vi "DMC VIDoc Confluence.vi"(8 "Error in":errorcluster caption="Error in (no error)") -> ()   [LabVIEW 2023]
uses:
  Git Type.ctl
  DMC CLI Confluence Documentation State.ctl
  <vilib>/Wiresmith Technology/G CLI/CLI Class/CLI.lvclass
  <vilib>/DMC/VIDoc/Printers/Confluence/Confluence Printer/Types/File Change Map.ctl
  Confluence Settings.ctl
  <vilib>/DMC/VIDoc/Framework/Parsing/TypeDefs/Full Documentation Info.ctl
  <vilib>/DMC/VIDoc/Framework/Parsing/Project Documentation/Project Documentation.lvclass
  <vilib>/DMC/VIDoc/Framework/Parsing/Interface Documenation/Interface Documenation.lvclass
  <vilib>/DMC/VIDoc/Framework/Parsing/Class Documentation/Class Documentation.lvclass
  <vilib>/DMC/VIDoc/Framework/Parsing/Library Documentation/Library Documentation.lvclass
  <vilib>/DMC/VIDoc/Framework/Parsing/GUI Documentation/GUI Documentation.lvclass
  <vilib>/DMC/VIDoc/Framework/Parsing/LLB Documentation/LLB Documentation.lvclass
  <vilib>/Wiresmith Technology/G CLI/Argument Parser/Option Class/Option Configuration.ctl
  <vilib>/Wiresmith Technology/G CLI/Argument Parser/Option Class/Argument Type.ctl
  8042783b-93c0-44c7-9b89-4fb89b10c9de.vi
  g-CLI Interaction/g-CLI Interaction.lvclass
  C:/Program Files/National Instruments/LabVIEW 2023/vi.lib/DMC/VIDoc/Framework/UI Interaction/Interface/UI Interaction.lvclass
  <vilib>/DMC/VIDoc/Printers/Confluence/Confluence Printer/VIDoc Printer - Confluence.lvclass
  <vilib>/Wiresmith Technology/G CLI/Argument Parser/Option Set Class/Option Set.lvclass
  <vilib>/Wiresmith Technology/G CLI/Argument Parser/Option Class/Option.lvclass
  <vilib>/DMC/VIDoc/Framework/Parsing/Documentation Parser/VIDoc Parser.lvclass
  <vilib>/DMC/VIDoc/Framework/Parsing/VIDoc Parsing.lvlib
panel:
  out "Scoped Token?":bool
  out "Confluence Token":string
  out "Confluence Email":string
  out "Confluence URL":string
  out "Use Data Center for Confluence Connection?":bool
  out "Use Login INI file for Confluence Connection?":bool
  out "Use Settings file for Confluence Connection Settings?":bool
  out "Top Page ID":string
  out "Source Paths":path[](array[path])
  out "Git Type":T1
  out "Run Git History?":bool
  out "Doc Settings Path":path
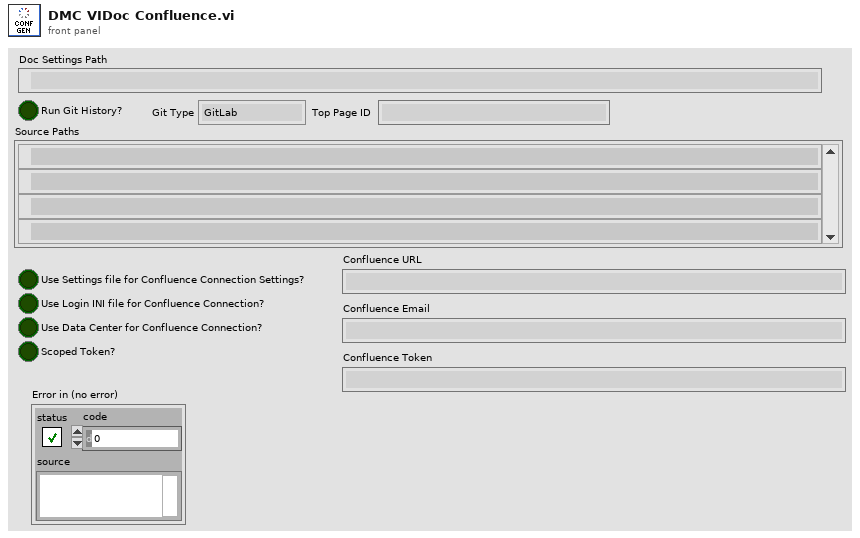
[diagram p1: front panel]
types:
  T1 = typedef "Git Type.ctl" = enum16{"GitLab", "GitHub", "BitBucket"}
  T2 = typedef "VIDoc Printer - Confluence.lvlib/VIDoc Printer - Confluence.lvclass/File Change Map.ctl" = map{string, cluster{"Timestamp":timestamp, "Commit Hash":string, "Author Name":string, "Branch":string, "Commit Hash URL":string}}
  T3 = typedef "Confluence Settings.ctl" = cluster{"Use INI?":bool, "URL":string, "Email":string, "Token":string, "Use Settings File?":bool, "Data Center?":bool, "Scoped Token?":bool}
  T4 = typedef "VIDoc Parsing.lvlib/Full Documentation Info.ctl" = cluster{"Projects":refnum<class "Project Documentation.lvclass">[], "Interfaces":refnum<class "Interface Documenation.lvclass">[], "Classes":refnum<class "Class Documentation.lvclass">[], "Libraries":refnum<class "Library Documentation.lvclass">[], "VI Members":refnum<class "GUI Documentation.lvclass">[], "Controls":refnum<class "GUI Documentation.lvclass">[], "LLBs":refnum<class "LLB Documentation.lvclass">[], "Bookmarked Map":map{string, refnum<class "GUI Documentation.lvclass">[]}}
  T5 = cluster{"CLI":refnum<class "CLI.lvclass">, "Working Directory":path, "Doc Settings Path":path, "Git History?":bool, "Git Type":T1, "File Change Map":T2, "Source Paths":path[], "Top Page ID":string, "Confluence Settings":T3, "Full Documentation":T4}
  T6 = typedef "DMC CLI Confluence Documentation State.ctl" = enum16{"Initialize", "Display Settings", "Git History", "Fetch Documentation", "Create Documentation", "Close", "Help"}
  T7 = enum16{"Doc Settings Path", "Git History", "Git Type", "Source Rel Paths", "Top Page ID", "Confluence Use Settings", "Confluence Use INI", "Confluence Type", "Confluence URL", "Confluence Email", "Confluence Token", "Scoped Token"}
  T8 = typedef "Option Parser.lvlib/Option.lvclass/Option Configuration.ctl" = cluster{"Option Type":T9, "Option Labels":string[], "Key":string, "Description":string, "Required":bool, "Default Value":string}
  T9 = typedef "Option Parser.lvlib/Option.lvclass/Argument Type.ctl" = enum16{"flag", "value"}
  T10 = enum16{"Doc Settings Path", "Git History", "Git Type", "Source Rel Paths", "Top Page ID", "Confluence Use Settings", "Confluence Use INI", "Confluence Type", "Confluence URL", "Confluence Email", "Confluence Token", "Scoped Token"}[]
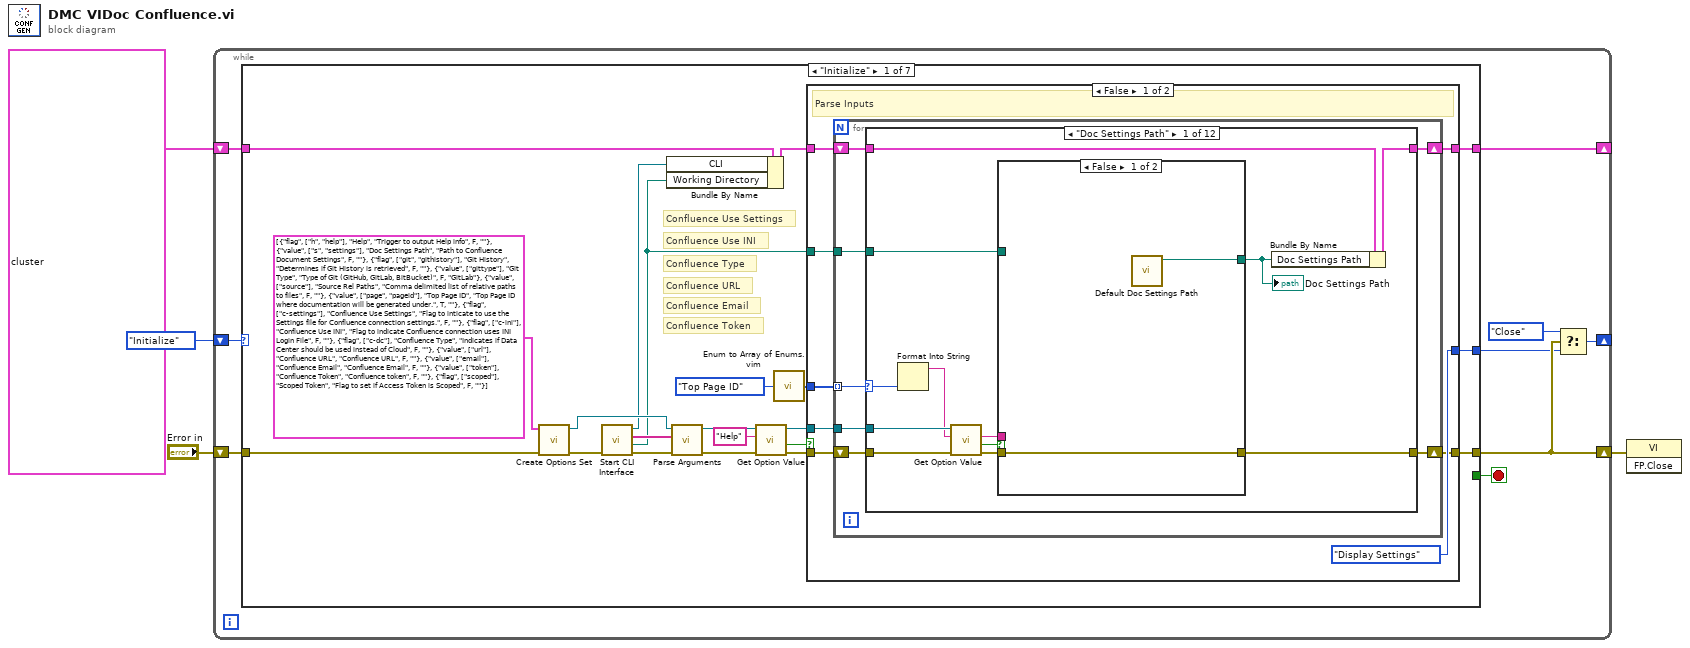
[diagram p0: block diagram]
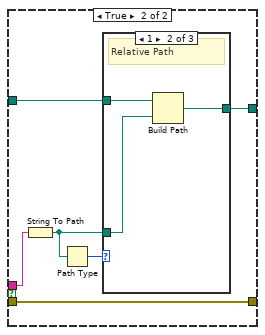
[diagram p2: hidden frame]
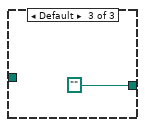
[diagram p4: hidden frame]
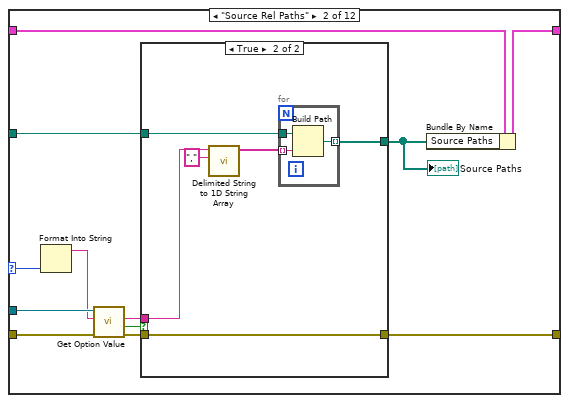
[diagram p5: hidden frame]
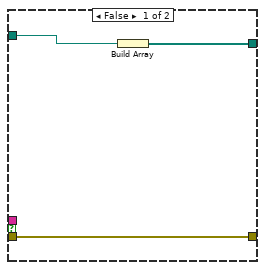
[diagram p6: hidden frame]
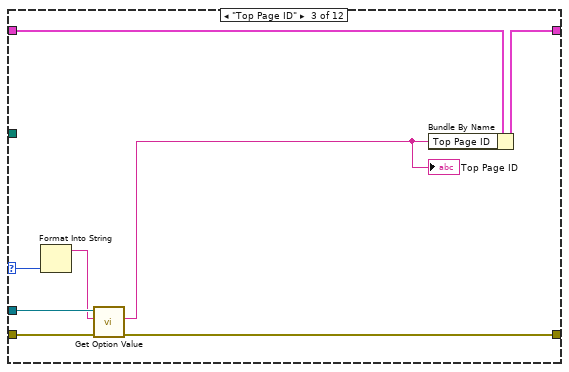
[diagram p7: hidden frame]
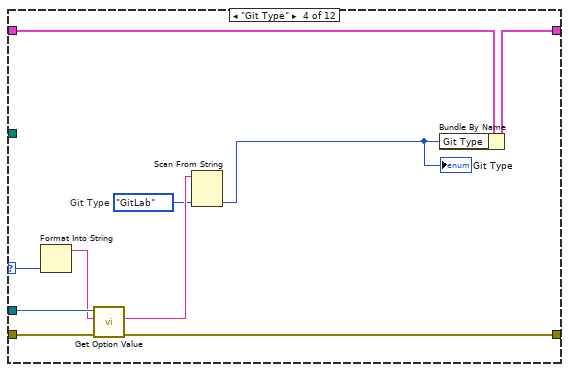
[diagram p8: hidden frame]
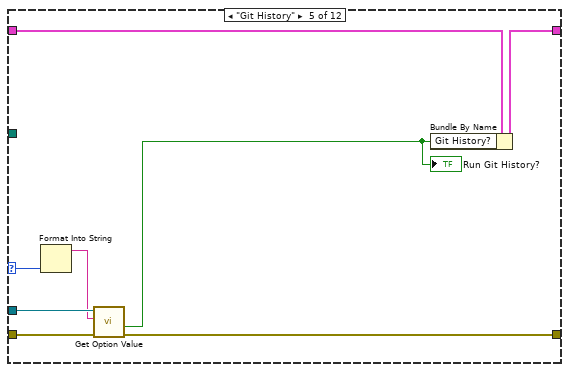
[diagram p9: hidden frame]
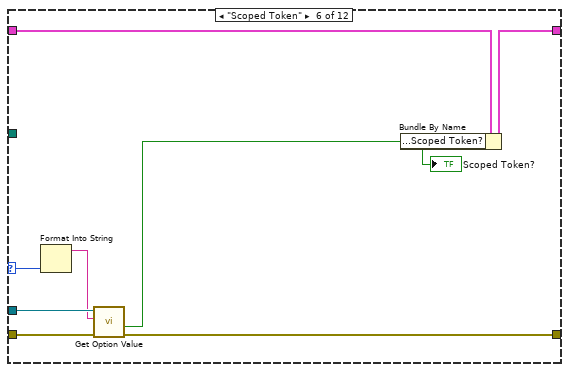
[diagram p10: hidden frame]
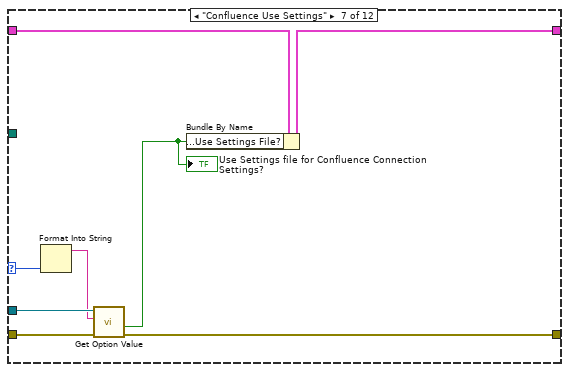
[diagram p11: hidden frame]
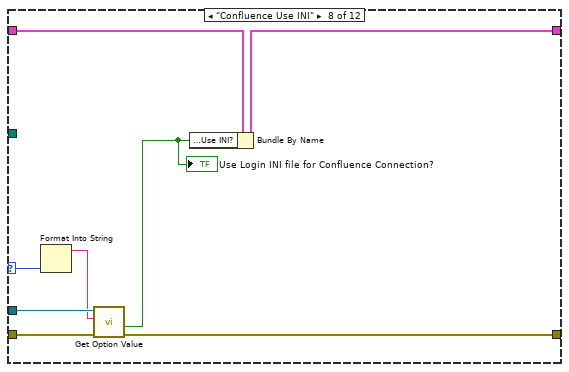
[diagram p12: hidden frame]
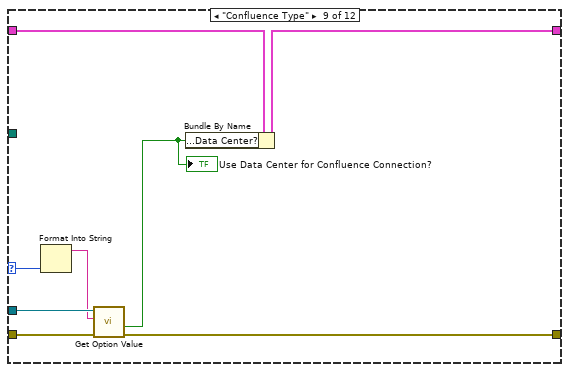
[diagram p13: hidden frame]
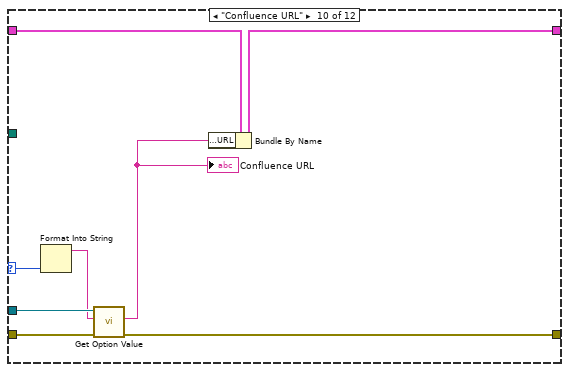
[diagram p14: hidden frame]
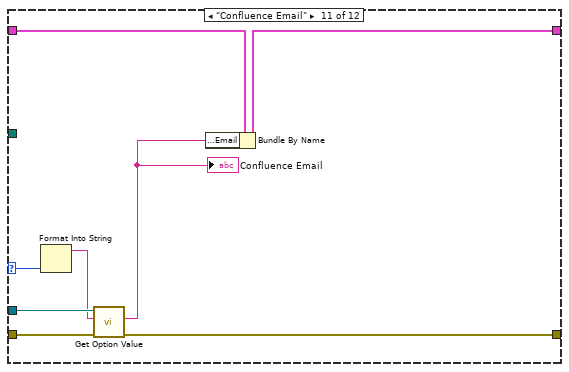
[diagram p15: hidden frame]
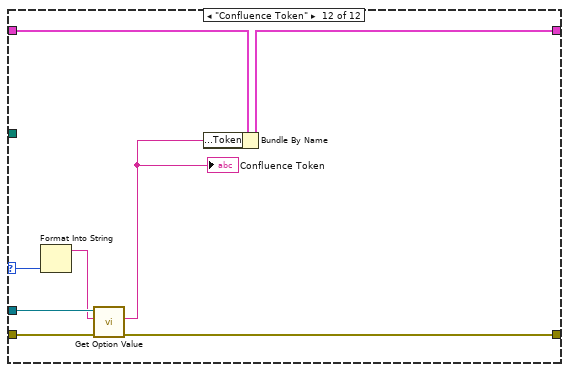
[diagram p16: hidden frame]
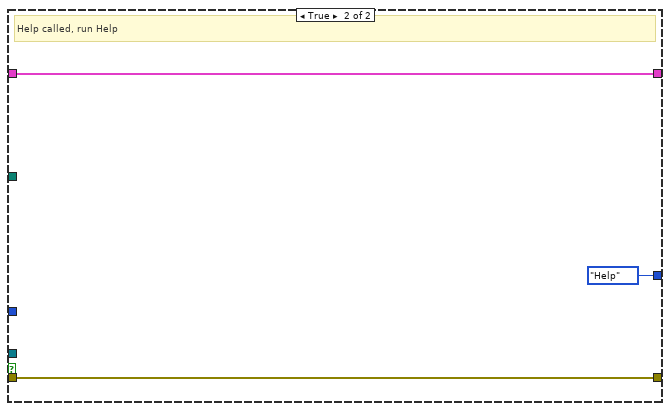
[diagram p17: hidden frame]
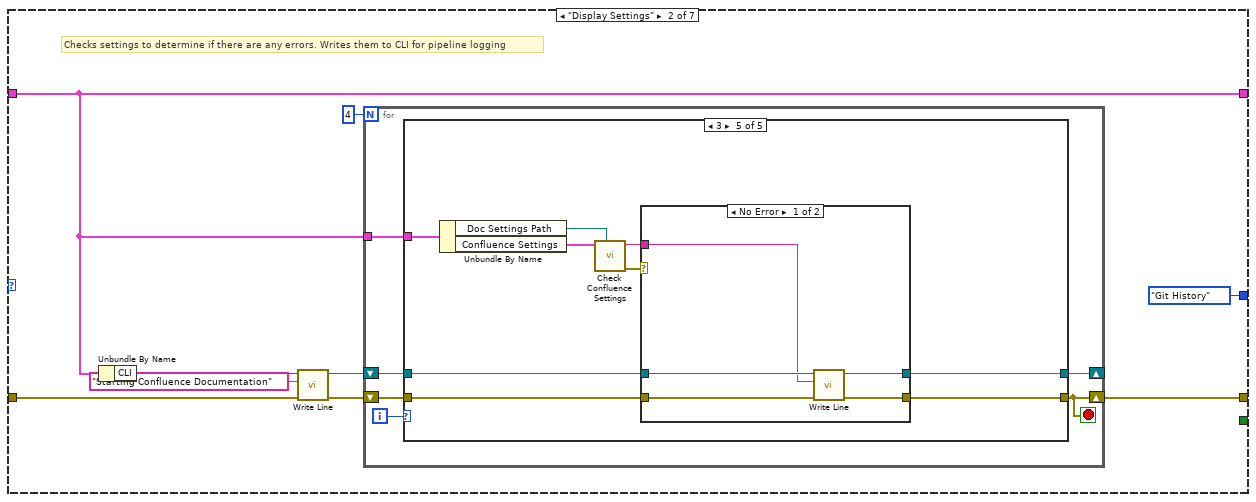
[diagram p18: hidden frame]
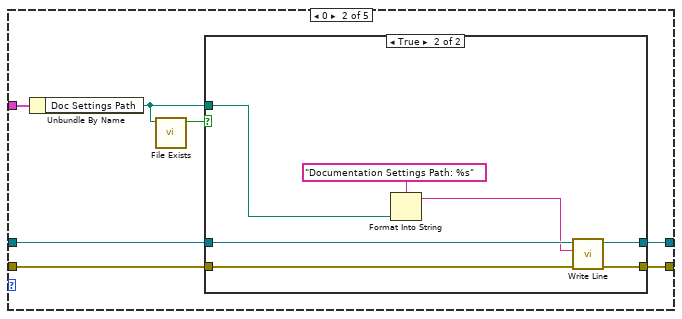
[diagram p20: hidden frame]
diagram:
  n1 = while {
    shift-right: [w8] -> _
    shift-left: DMC_CLI_Confluence_Documentation_State."Initialize" -> [w13]
    shift-right: [w10] -> w1
    shift-left: "Error in" -> [w12]
    shift-right: [w5] -> _
    shift-left: T5 {"CLI"=refnum, "Working Directory"=path "", "Doc Settings Path"=path "", "Git History?"=FALSE, "Git Type"=enum."GitLab", "File Change Map"={}, "Source Paths"=[], "Top Page ID"="", "Confluence Settings"={"Use INI?"=FALSE, "URL"="", "Email"="", "Token"="", "Use Settings File?"=FALSE, "Data Center?"=FALSE, "Scoped Token?"=FALSE}, "Full Documentation"={"Projects"=[], "Interfaces"=[], "Classes"=[], "Libraries"=[], "VI Members"=[], "Controls"=[], "LLBs"=[], "Bookmarked Map"={}}} -> [w6]
    stop <- w7 stop-if-true
    n2 = case shown="\"Initialize\"" w13 {
      tunnel: w12 -> [w26 w187 w272 w308 w322 w334 w344]
      tunnel: [w17 w192 w269 w292 w324 w335 w345] -> w10
      tunnel: [w19 DMC_CLI_Confluence_Documentation_State."Git History" DMC_CLI_Confluence_Documentation_State."Fetch Documentation" DMC_CLI_Confluence_Documentation_State."Create Documentation" DMC_CLI_Confluence_Documentation_State."Close" DMC_CLI_Confluence_Documentation_State."Close" DMC_CLI_Confluence_Documentation_State."Close"] -> w9
      tunnel: [_ _ _ _ _ TRUE _] -> w7
      tunnel: w6 -> [w25 w191 w270 w309 w323 w338 w342]
      tunnel: [w21 w191 w271 w303 w323 w338 w342] -> w5
      frame "Initialize" {
        # "Confluence Token"
        # "Confluence Email"
        # "Confluence URL"
        # "Confluence Type"
        # "Confluence Use INI"
        # "Confluence Use Settings"
        n3 = call <vilib>:"Create Options Set.vi"("error in (no error)"=w26, "Options"=T8[] [{"Option Type"=enum."flag", "Option Labels"=["h", "help"], "Key"="Help", "Description"="Trigger to output Help info", "Required"=FALSE, "Default Value"=""}, {"Option Type"=enum."value", "Option Labels"=["s", "settings"], "Key"="Doc Settings Path", "Description"="Path to Confluence Document Settings", "Required"=FALSE, "Default Value"=""}, {"Option Type"=enum."flag", "Option Labels"=["git", "githistory"], "Key"="Git History", "Description"="Determines if Git History is retrieved", "Required"=FALSE, "Default Value"=""}, {"Option Type"=enum."value", "Option Labels"=["gittype"], "Key"="Git Type", "Description"="Type of Git (GitHub, GitLab, BitBucket)", "Required"=FALSE, "Default Value"="GitLab"}, {"Option Type"=enum."value", "Option Labels"=["source"], "Key"="Source Rel Paths", "Description"="Comma delimited list of relative paths to files", "Required"=FALSE, "Default Value"=""}, {"Option Type"=enum."value", "Option Labels"=["page", "pageid"], "Key"="Top Page ID", "Description"="Top Page ID where documentation will be generated under.", "Required"=TRUE, "Default Value"=""}, {"Option Type"=enum."flag", "Option Labels"=["c-settings"], "Key"="Confluence Use Settings", "Description"="Flag to inticate to use the Settings file for Confluence connection settings.", "Required"=FALSE, "Default Value"=""}, {"Option Type"=enum."flag", "Option Labels"=["c-ini"], "Key"="Confluence Use INI", "Description"="Flag to indicate Confluence connection uses INI Login File", "Required"=FALSE, "Default Value"=""}, {"Option Type"=enum."flag", "Option Labels"=["c-dc"], "Key"="Confluence Type", "Description"="Indicates if Data Center should be used instead of Cloud", "Required"=FALSE, "Default Value"=""}, {"Option Type"=enum."value", "Option Labels"=["url"], "Key"="Confluence URL", "Description"="Confluence URL", "Required"=FALSE, "Default Value"=""}, {"Option Type"=enum."value", "Option Labels"=["email"], "Key"="Confluence Email", "Description"="Confluence Email", "Required"=FALSE, "Default Value"=""}, {"Option Type"=enum."value", "Option Labels"=["token"], "Key"="Confluence Token", "Description"="Confluence token", "Required"=FALSE, "Default Value"=""}, {"Option Type"=enum."flag", "Option Labels"=["scoped"], "Key"="Scoped Token", "Description"="Flag to set if Access Token is Scoped", "Required"=FALSE, "Default Value"=""}]) -> ("error out"=w32:errorcluster, "Option Set out"=w31:refnum<class "Option Set.lvclass">)  [unwired: 8 in]
        n4 = call <vilib>:"Start CLI Interface.vi"("error in (no error)"=w32) -> ("error out"=w34:errorcluster, "Working Directory"=w14:path, "Custom Parameters"=w30:string[], "CLI out"=w24:refnum<class "CLI.lvclass">)  [unwired: 7 in]
        n5 = Bundle By Name(cluster=w25, "CLI"=w24, "Working Directory"=w14) -> (w20:T5)
        n6 = call <vilib>:"Parse Arguments.vi"("error in (no error)"=w34, "Arguments"=w30, "Option Set in"=w31) -> ("error out"=w28:errorcluster, "Option Set out"=w27:refnum<class "Option Set.lvclass">)  [unwired: 5 in, 2 out]
        n7 = call <vilib>:"Get Option Value.vi"("error in (no error)"=w28, "Option Key"="Help", "Option Set in"=w27) -> ("error out"=w18:errorcluster, "Set"=w23:bool, "Option Set out"=w22:refnum<class "Option Set.lvclass">)  [unwired: 5 in, 1 out]
        n8 = call "Enum to Array of Enums.vim"("enum"=T7."Top Page ID") -> ("array of enums"=w15:T10)
        n9 = case shown="False" w23 {
          tunnel: w22 -> [w41 _]
          tunnel: [w39 w183] -> w21
          tunnel: w20 -> [w40 w183]
          tunnel: [DMC_CLI_Confluence_Documentation_State."Display Settings" DMC_CLI_Confluence_Documentation_State."Help"] -> w19
          tunnel: w18 -> [w42 w181]
          tunnel: [w35 w181] -> w17
          tunnel: w15 -> [w38 _]
          tunnel: w14 -> [w37 _]
          frame False {
            # "Parse Inputs"
            n10 = for {
              shift-right: [w44] -> w35
              shift-left: w42 -> [w45]
              tunnel: w41 -> [w46]
              shift-right: [w47] -> w39
              shift-left: w40 -> [w48]
              tunnel: w38 -> [w49] mode=indexing
              tunnel: w37 -> [w43]
              n11 = case shown="\"Doc Settings Path\"" w49 {
                selector: w49 -> [w58 w83 w103 w113 w121 w129 w137 w145 w153 w161 w169 w177]
                tunnel: w48 -> [w61 w86 w106 w116 w124 w132 w140 w148 w156 w164 w172 w180]
                tunnel: [w52 w77 w100 w111 w118 w126 w134 w142 w150 w158 w166 w174] -> w47
                tunnel: w46 -> [w59 w84 w104 w114 w122 w130 w138 w146 w154 w162 w170 w178]
                tunnel: w45 -> [w60 w85 w105 w115 w123 w131 w139 w147 w155 w163 w171 w179]
                tunnel: [w53 w78 w101 w107 w119 w127 w135 w143 w151 w159 w167 w175] -> w44
                tunnel: w43 -> [w50 w75 _ _ _ _ _ _ _ _ _ _]
                frame "Doc Settings Path" {
                  n12 = Format Into String(w58) -> (resulting string=w57:string)  [unwired: 3 in, 1 out]
                  n13 = call <vilib>:"Get Option Value.vi"("error in (no error)"=w60, "Option Key"=w57, "Option Set in"=w59) -> ("error out"=w56:errorcluster, "Set"=w54:bool, "Value"=w55:string)  [unwired: 5 in, 1 out]
                  n14 = case shown="False" w54 {
                    tunnel: w56 -> [w62 w69]
                    tunnel: w55 -> [_ w68]
                    tunnel: [w62 w69] -> w53
                    tunnel: [w63 w65] -> w51
                    tunnel: w50 -> [_ w64]
                    frame False {
                      n15 = call "Default Doc Settings Path.vi"() -> ("Default Doc Settings Path"=w63:path)  [unwired: 11 in]
                    }
                    frame True {
                      n16 = String To Path(string=w68) -> (path=w66:path)
                      n17 = Path Type(1:w66) -> (0:w67:i16)
                      n18 = case shown="1" w67 {
                        tunnel: w66 -> [w70 w72 _]
                        tunnel: [w70 w71 path ""] -> w65
                        tunnel: w64 -> [_ w73 _]
                        frame 0 {
                          # "Absolute Path"
                        }
                        frame 1 {
                          # "Relative Path"
                          n19 = Build Path(base path=w73, name or relative path=w72) -> (appended path=w71:path)
                        }
                        frame Default {
                        }
                      }
                    }
                  }
                  "Doc Settings Path" <- w51
                  n20 = Bundle By Name(cluster=w61, "Doc Settings Path"=w51) -> (w52:T5)
                }
                frame "Source Rel Paths" {
                  n21 = Format Into String(w83) -> (resulting string=w82:string)  [unwired: 3 in, 1 out]
                  n22 = call <vilib>:"Get Option Value.vi"("error in (no error)"=w85, "Option Key"=w82, "Option Set in"=w84) -> ("error out"=w81:errorcluster, "Set"=w79:bool, "Value"=w80:string)  [unwired: 5 in, 1 out]
                  n23 = case shown="True" w79 {
                    tunnel: w81 -> [w89 w95]
                    tunnel: w80 -> [_ w94]
                    tunnel: [w89 w95] -> w78
                    tunnel: [w87 w92] -> w76
                    tunnel: w75 -> [w88 w91]
                    frame False {
                      n24 = Build Array(w88) -> (w87:path[])
                    }
                    frame True {
                      n25 = call <vilib>:"Delimited String to 1D String Array.vi"("delimiter"=",", "delimited string"=w94) -> ("string array"=w90:string[])  [unwired: 9 in]
                      n26 = for {
                        tunnel: w91 -> [w98]
                        tunnel: w90 -> [w97] mode=indexing
                        tunnel: [w96] -> w92 mode=indexing
                        n27 = Build Path(base path=w98, name or relative path=w97) -> (appended path=w96:path)
                      }
                    }
                  }
                  "Source Paths" <- w76
                  n28 = Bundle By Name(cluster=w86, "Source Paths"=w76) -> (w77:T5)
                }
                frame "Top Page ID" {
                  n29 = Format Into String(w103) -> (resulting string=w102:string)  [unwired: 3 in, 1 out]
                  n30 = call <vilib>:"Get Option Value.vi"("error in (no error)"=w105, "Option Key"=w102, "Option Set in"=w104) -> ("error out"=w101:errorcluster, "Value"=w99:string)  [unwired: 5 in, 2 out]
                  "Top Page ID" <- w99
                  n31 = Bundle By Name(cluster=w106, "Top Page ID"=w99) -> (w100:T5)
                }
                frame "Git Type" {
                  w109 = Git_Type."GitLab"  # Git Type
                  n32 = Format Into String(w113) -> (resulting string=w112:string)  [unwired: 3 in, 1 out]
                  n33 = call <vilib>:"Get Option Value.vi"("error in (no error)"=w115, "Option Key"=w112, "Option Set in"=w114) -> ("error out"=w107:errorcluster, "Value"=w110:string)  [unwired: 5 in, 2 out]
                  n34 = Scan From String(input string=w110, default 1=w109) -> (output 1=w108:T1)  [unwired: 3 in, 3 out]
                  "Git Type" <- w108
                  n35 = Bundle By Name(cluster=w116, "Git Type"=w108) -> (w111:T5)
                }
                frame "Git History" {
                  n36 = Format Into String(w121) -> (resulting string=w120:string)  [unwired: 3 in, 1 out]
                  n37 = call <vilib>:"Get Option Value.vi"("error in (no error)"=w123, "Option Key"=w120, "Option Set in"=w122) -> ("error out"=w119:errorcluster, "Set"=w117:bool)  [unwired: 5 in, 2 out]
                  "Run Git History?" <- w117
                  n38 = Bundle By Name(cluster=w124, "Git History?"=w117) -> (w118:T5)
                }
                frame "Scoped Token" {
                  n39 = Format Into String(w129) -> (resulting string=w128:string)  [unwired: 3 in, 1 out]
                  n40 = call <vilib>:"Get Option Value.vi"("error in (no error)"=w131, "Option Key"=w128, "Option Set in"=w130) -> ("error out"=w127:errorcluster, "Set"=w125:bool)  [unwired: 5 in, 2 out]
                  "Scoped Token?" <- w125
                  n41 = Bundle By Name(cluster=w132, "Confluence Settings.Scoped Token?"=w125) -> (w126:T5)
                }
                frame "Confluence Use Settings" {
                  n42 = Format Into String(w137) -> (resulting string=w136:string)  [unwired: 3 in, 1 out]
                  n43 = call <vilib>:"Get Option Value.vi"("error in (no error)"=w139, "Option Key"=w136, "Option Set in"=w138) -> ("error out"=w135:errorcluster, "Set"=w133:bool)  [unwired: 5 in, 2 out]
                  "Use Settings file for Confluence Connection Settings?" <- w133
                  n44 = Bundle By Name(cluster=w140, "Confluence Settings.Use Settings File?"=w133) -> (w134:T5)
                }
                frame "Confluence Use INI" {
                  n45 = Format Into String(w145) -> (resulting string=w144:string)  [unwired: 3 in, 1 out]
                  n46 = call <vilib>:"Get Option Value.vi"("error in (no error)"=w147, "Option Key"=w144, "Option Set in"=w146) -> ("error out"=w143:errorcluster, "Set"=w141:bool)  [unwired: 5 in, 2 out]
                  "Use Login INI file for Confluence Connection?" <- w141
                  n47 = Bundle By Name(cluster=w148, "Confluence Settings.Use INI?"=w141) -> (w142:T5)
                }
                frame "Confluence Type" {
                  n48 = Format Into String(w153) -> (resulting string=w152:string)  [unwired: 3 in, 1 out]
                  n49 = call <vilib>:"Get Option Value.vi"("error in (no error)"=w155, "Option Key"=w152, "Option Set in"=w154) -> ("error out"=w151:errorcluster, "Set"=w149:bool)  [unwired: 5 in, 2 out]
                  "Use Data Center for Confluence Connection?" <- w149
                  n50 = Bundle By Name(cluster=w156, "Confluence Settings.Data Center?"=w149) -> (w150:T5)
                }
                frame "Confluence URL" {
                  n51 = Format Into String(w161) -> (resulting string=w160:string)  [unwired: 3 in, 1 out]
                  n52 = call <vilib>:"Get Option Value.vi"("error in (no error)"=w163, "Option Key"=w160, "Option Set in"=w162) -> ("error out"=w159:errorcluster, "Value"=w157:string)  [unwired: 5 in, 2 out]
                  "Confluence URL" <- w157
                  n53 = Bundle By Name(cluster=w164, "Confluence Settings.URL"=w157) -> (w158:T5)
                }
                frame "Confluence Email" {
                  n54 = Format Into String(w169) -> (resulting string=w168:string)  [unwired: 3 in, 1 out]
                  n55 = call <vilib>:"Get Option Value.vi"("error in (no error)"=w171, "Option Key"=w168, "Option Set in"=w170) -> ("error out"=w167:errorcluster, "Value"=w165:string)  [unwired: 5 in, 2 out]
                  "Confluence Email" <- w165
                  n56 = Bundle By Name(cluster=w172, "Confluence Settings.Email"=w165) -> (w166:T5)
                }
                frame "Confluence Token" {
                  n57 = Format Into String(w177) -> (resulting string=w176:string)  [unwired: 3 in, 1 out]
                  n58 = call <vilib>:"Get Option Value.vi"("error in (no error)"=w179, "Option Key"=w176, "Option Set in"=w178) -> ("error out"=w175:errorcluster, "Value"=w173:string)  [unwired: 5 in, 2 out]
                  "Confluence Token" <- w173
                  n59 = Bundle By Name(cluster=w180, "Confluence Settings.Token"=w173) -> (w174:T5)
                }
              }
            }
          }
          frame True {
            # "Help called, run Help"
          }
        }
      }
      frame "Display Settings" {
        # "Checks settings to determine if there are any errors. Writes them to CLI for pipeline logging"
        n60 = Unbundle By Name(w191) -> ("CLI"=w188:refnum<class "CLI.lvclass">)
        n61 = call <vilib>:"Write Line.vi"("error in (no error)"=w187, "Text to Write"="Starting Confluence Documentation", "CLI in"=w188) -> ("error out"=w186:errorcluster, "CLI out"=w185:refnum<class "CLI.lvclass">)  [unwired: 7 in]
        n62 = for {
          N: 4 -> [_]
          shift-right: [w193] -> w192
          shift-left: w186 -> [w197]
          shift-right: [w196] -> _
          shift-left: w185 -> [w198]
          tunnel: w191 -> [w194]
          i -> [w195]
          stop <- w193 stop-if-true
          n63 = case shown="3" w195 {
            tunnel: w198 -> [w199 w207 w232 w239 w256]
            tunnel: [w200 w206 w231 w238 w255] -> w193
            tunnel: w197 -> [w200 w205 w230 w237 w257]
            tunnel: [w199 w204 w229 w236 w254] -> w196
            tunnel: w194 -> [_ w203 w228 w235 w260]
            frame Default {
            }
            frame 0 {
              n64 = Unbundle By Name(w203) -> ("Doc Settings Path"=w202:path)
              n65 = call "File Exists.vi"("Path"=w202) -> ("Exists?"=w201:bool)  [unwired: 9 in, 1 out]
              n66 = case shown="True" w201 {
                tunnel: w207 -> [w214 w221]
                tunnel: [w212 w220] -> w206
                tunnel: w205 -> [w213 w219]
                tunnel: [w214 w218] -> w204
                tunnel: w202 -> [w209 w216]
                frame False {
                  n67 = Format Into String(format string="Documentation Settings File Doesn't Exist: %s", w209) -> (resulting string=w208:string)  [unwired: 2 in, 1 out]
                  n68 = call <vilib>:"Error Cluster From Error Code.vi"("error in (no error)"=w213, "error message (\"\")"=w208, "error code (0)"=5555) -> ("error out"=w212:errorcluster)  [unwired: 6 in]
                }
                frame True {
                  n69 = Format Into String(format string="Documentation Settings Path: %s", w216) -> (resulting string=w215:string)  [unwired: 2 in, 1 out]
                  n70 = call <vilib>:"Write Line.vi"("error in (no error)"=w219, "Text to Write"=w215, "CLI in"=w221) -> ("error out"=w220:errorcluster, "CLI out"=w218:refnum<class "CLI.lvclass">)  [unwired: 7 in]
                }
              }
            }
            frame 1 {
              n71 = Unbundle By Name(w228) -> ("Source Paths"=w225:path[])
              n72 = Path To String(path=w225) -> (string=w224:string[])
              n73 = call <vilib>:"1D String Array to Delimited String.vi"("delimiter"="\r\n", "string array"=w224) -> ("delimited string"=w222:string)  [unwired: 9 in]
              n74 = Format Into String(format string="Source Paths: %s", w222) -> (resulting string=w226:string)  [unwired: 2 in, 1 out]
              n75 = call <vilib>:"Write Line.vi"("error in (no error)"=w230, "Text to Write"=w226, "CLI in"=w232) -> ("error out"=w231:errorcluster, "CLI out"=w229:refnum<class "CLI.lvclass">)  [unwired: 7 in]
            }
            frame 2 {
              n76 = Unbundle By Name(w235) -> ("Top Page ID"=w234:string)
              n77 = Empty String/Path?(string/path=w234) -> (empty?=w233:bool)
              n78 = case shown="False" w233 {
                tunnel: w239 -> [w246 w251]
                tunnel: [w245 w249] -> w238
                tunnel: w237 -> [w244 w250]
                tunnel: [w243 w251] -> w236
                tunnel: w234 -> [w240 _]
                frame False {
                  n79 = Format Into String(format string="Top Page ID: %s", w240) -> (resulting string=w241:string)  [unwired: 2 in, 1 out]
                  n80 = call <vilib>:"Write Line.vi"("error in (no error)"=w244, "Text to Write"=w241, "CLI in"=w246) -> ("error out"=w245:errorcluster, "CLI out"=w243:refnum<class "CLI.lvclass">)  [unwired: 7 in]
                }
                frame True {
                  n81 = call <vilib>:"Error Cluster From Error Code.vi"("error in (no error)"=w250, "error message (\"\")"="No Top Page ID Assigned." ("error message (\"\")"), "error code (0)"=5556) -> ("error out"=w249:errorcluster)  [unwired: 6 in]
                }
              }
            }
            frame 3 {
              n82 = Unbundle By Name(w260) -> ("Doc Settings Path"=w259:path, "Confluence Settings"=w258:T3)
              n83 = call "Check Confluence Settings.vi"("Settings Path"=w259, "Confluence Settings"=w258) -> ("Error out"=w252:errorcluster, "String"=w253:string)  [unwired: 8 in]
              n84 = case shown="No Error" w252 {
                selector: w252 -> [_ w267]
                tunnel: w257 -> [w265 _]
                tunnel: w256 -> [w264 w266]
                tunnel: [w263 w267] -> w255
                tunnel: [w262 w266] -> w254
                tunnel: w253 -> [w261 _]
                frame No Error {
                  n85 = call <vilib>:"Write Line.vi"("error in (no error)"=w265, "Text to Write"=w261, "CLI in"=w264) -> ("error out"=w263:errorcluster, "CLI out"=w262:refnum<class "CLI.lvclass">)  [unwired: 7 in]
                }
                frame Error {
                }
              }
            }
          }
        }
      }
      frame "Git History" {
        n86 = Unbundle By Name(w270) -> ("Git History?"=w273:bool)
        n87 = case shown="True" w273 {
          tunnel: w272 -> [w275 w291]
          tunnel: [w274 w283] -> w271
          tunnel: w270 -> [w274 w284]
          tunnel: [w275 w280] -> w269
          frame False {
          }
          frame True {
            n88 = Unbundle By Name(w284) -> ("Git Type"=w286:T1, "Working Directory"=w287:path, "CLI"=w290:refnum<class "CLI.lvclass">)
            n89 = call <vilib>:"Write Line.vi"("error in (no error)"=w291, "Text to Write"="Loading Git History", "CLI in"=w290) -> ("error out"=w288:errorcluster, "CLI out"=w279:refnum<class "CLI.lvclass">)  [unwired: 7 in]
            n90 = call "Git History.vi"("Git Type"=w286, "Error in"=w288, "Branch Hierarchy"=string[] ["master", "main", "dev", "feature", "hot-fix"], "Working Directory"=w287) -> ("Error out"=w281:errorcluster, "File Change Map"=w282:T2)  [unwired: 6 in]
            n91 = Collection Size(1:w282) -> (0:w277:i32)
            n92 = Format Into String(format string="Read Git History: %d Files", w277) -> (resulting string=w276:string)  [unwired: 2 in, 1 out]
            n93 = call <vilib>:"Write Line.vi"("error in (no error)"=w281, "Text to Write"=w276, "CLI in"=w279) -> ("error out"=w280:errorcluster)  [unwired: 7 in, 1 out]
            n94 = Bundle By Name(cluster=w284, "File Change Map"=w282) -> (w283:T5)
          }
        }
      }
      frame "Fetch Documentation" {
        n95 = Unbundle By Name(w309) -> ("Source Paths"=w296:path[], "Doc Settings Path"=w299:path, "CLI"=w307:refnum<class "CLI.lvclass">)
        n96 = call <vilib>:"Write Line.vi"("error in (no error)"=w308, "Text to Write"="Parsing Source Files", "CLI in"=w307) -> ("error out"=w305:errorcluster, "CLI out"=w304:refnum<class "CLI.lvclass">)  [unwired: 7 in]
        n97 = call "Wrap g-CLI.vi"("error in (no error)"=w305, "CLI"=w304) -> ("error out"=w300:errorcluster, "g-CLI Interaction out"=w301:refnum<class "g-CLI Interaction.lvclass">)  [unwired: 8 in]
        n98 = call <vilib>:"Initialize.vi"("error in (no error)"=w300, "Settings Path"=w299, "UI Interaction"=w301) -> ("error out"=w297:errorcluster, "VIDoc Parser Out"=w298:refnum<class "VIDoc Parser.lvclass">)  [unwired: 7 in]
        n99 = call <vilib>:"Fetch Full Documentation.vi"("error in (no error)"=w297, "File Paths"=w296, "VIDoc Parser In"=w298) -> ("error out"=w294:errorcluster, "Full Documentation"=w295:T4, "VIDoc Parser Out"=w293:refnum<class "VIDoc Parser.lvclass">)  [unwired: 6 in]
        n100 = call <vilib>:"Close.vi"("error in (no error)"=w294, "VIDoc Parser In"=w293) -> ("error out"=w292:errorcluster)  [unwired: 9 in]
        n101 = Bundle By Name(cluster=w309, "Full Documentation"=w295) -> (w303:T5)
      }
      frame "Create Documentation" {
        n102 = Unbundle By Name(w323) -> ("Full Documentation"=w319:T4, "Doc Settings Path"=w320:path, "Top Page ID"=w315:string, "Working Directory"=w316:path, "File Change Map"=w317:T2, "Confluence Settings"=w311:T3, "CLI"=w310:refnum<class "CLI.lvclass">)
        n103 = call "Wrap g-CLI.vi"("error in (no error)"=w322, "CLI"=w310) -> ("error out"=w314:errorcluster, "g-CLI Interaction out"=w321:refnum<class "g-CLI Interaction.lvclass">)  [unwired: 8 in]
        n104 = call "Determine Confluence Connection.vi"("Error in"=w314, "Confluence Settings"=w311) -> ("Error out"=w313:errorcluster, "Confluence"=w312:refnum<class "Confluence.lvclass">)  [unwired: 8 in]
        n105 = call <vilib>:"Construct.vi"("File Change Map"=w317, "error in (no error)"=w313, "Working Directory"=w316, "Top Page ID"=w315, "Confluence"=w312) -> ("error out"=w331:errorcluster, "VIDoc Printer - Confluence Out"=w332:refnum<class "VIDoc Printer - Confluence.lvclass">)  [unwired: 5 in]
        n106 = call-dynamic <vilib>:"Initialize.vi"("UI Interaction"=w321, "error in (no error)"=w331, "Settings Path"=w320, "VIDoc Printer - Confluence In"=w332) -> ("error out"=w329:errorcluster, "VIDoc Printer - Confluence Out"=w330:refnum<class "VIDoc Printer - Confluence.lvclass">)  [unwired: 6 in]
        n107 = call-dynamic "Report.vi"("error in (no error)"=w329, "Full Documentation"=w319, "VIDoc Printer In"=w330) -> ("error out"=w327:errorcluster, "VIDoc Printer Out"=w328:refnum<class "VIDoc Printer - Confluence.lvclass">)  [unwired: 7 in]
        n108 = call <vilib>:"Publish Pages.vi"("error in (no error)"=w327, "VIDoc Printer - Confluence In"=w328) -> ("error out"=w325:errorcluster, "VIDoc Printer - Confluence Out"=w326:refnum<class "VIDoc Printer - Confluence.lvclass">)  [unwired: 8 in]
        n109 = call-dynamic <vilib>:"Close.vi"("error in (no error)"=w325, "VIDoc Printer - Confluence In"=w326) -> ("error out"=w324:errorcluster)  [unwired: 9 in]
      }
      frame "Close" {
        n110 = Unbundle By Name(w338) -> ("CLI"=w336:refnum<class "CLI.lvclass">)
        n111 = call <vilib>:"Write Line.vi"("Text to Write"="Exiting Confluence Documentation", "CLI in"=w336) -> ("CLI out"=w333:refnum<class "CLI.lvclass">)  [unwired: 8 in, 1 out]
        n112 = call <vilib>:"Exit With Error Cluster Code.vi"("error in (no error)"=w334, "CLI in"=w333) -> ("error out"=w335:errorcluster)  [unwired: 9 in]
      }
      frame "Help" {
        n113 = Unbundle By Name(w342) -> ("CLI"=w341:refnum<class "CLI.lvclass">)
        n114 = call <vilib>:"Write Line.vi"("error in (no error)"=w344, "Text to Write"="-------required arguments-------\n-pageid <Page ID for the top level Confluence Page that documentation will be generated under>\n\n-------optional arguments-------\n-settings <absolute or relative to working directory relative path to Doc Settings file. defaults to Default.json included with app>\n-git <Flag to include Git History in the documentation>\n-gittype <Indicates which Git repo type the Git History would check. Defaults to GitLab, also allows GitHub and BitBucket>\n-source <comma seperated string of all relative file paths within working directory to include. Recursive search. Defaults to whole working directory>\n-c-settings <Flag to indicate use the Confluence connection settings from within the Doc Settings File>\n-c-ini <Flag to indicate using the Login INI file for Confluence connections>\n-c-dc <Indicates Confluence type. If flag present then uses Data Center, otherwise uses Cloud>\n-url <Confluence URL>\n-email <Confluence Email>\n-token <Confluence Access Token>\n-scoped <Indicates if Access Token is Scoped or not>\n-help <Returns this help information>" ("string"), "CLI in"=w341) -> ("error out"=w345:errorcluster)  [unwired: 7 in, 1 out]
      }
    }
    n115 = Select(t=DMC_CLI_Confluence_Documentation_State."Close", s=w10, f=w9) -> (s? t:f=w8:T6)
  }
  n116 = invoke class="VI" method="FP.Close"(error in=w1) -> ()  [unwired: 2 in, 3 out]
